vi "Slave - Latency Bmk - Queue.vi"() -> ()   [LabVIEW 2016]
uses:
  <vilib>/Utility/error.llb/DialogType.ctl
  <vilib>/Analysis/baseanly.llb/Mean (DBL).vi
  <vilib>/pximc/Initialize Writer Session (DBL).vi
  <vilib>/pximc/Initialize Reader Session (DBL).vi
  <vilib>/pximc/Connect (DBL).vi
  <vilib>/pximc/Write (DBL).vi
  <vilib>/pximc/Read (DBL).vi
  <vilib>/pximc/nipximc.lvlib
  <vilib>/Analysis/NI_AALBase.lvlib
panel:
  out "size(s) 2":i32
  out "size(s)":i32
  out "Avg Elapsed Time 2":dbl
  out "Value Change Timestamp 2":u32 caption="Tick Count(uSec)"
  out "Instant Elapsed Time 2":i32
  out "Avg Elapsed Time":dbl
  out "Instant Elapsed Time":i32
  out "Value Change Timestamp":u32 caption="Tick Count(uSec)"
  in  "Node 1 Reader Connection ID":u16=4
  in  "Reader Interface Node 2":tag="PXIMC2" caption="interface"
  in  "Node 2 Writer Connection ID":u16=3
  in  "Writer Interface Node 2":tag="PXIMC2" caption="interface"
  out "Stopped?":bool
  in  "Node 1 Writer Connection ID":u16=1
  in  "Node 1 Writer Interface":tag="PXIMC2" caption="interface"
  in  "Stop Button":bool
  in  "Node 1 Reader Interface":tag="PXIMC2" caption="interface"
  in  "Buffer Size":u64=250000 caption="buffer size"
  in  "Connection Timeout (s)":dbl=60.0 caption="timeout in seconds (-1)"
  in  "Node 1 Reader Connection ID":u16=2
  # "Node 1"
  # "Node 2"
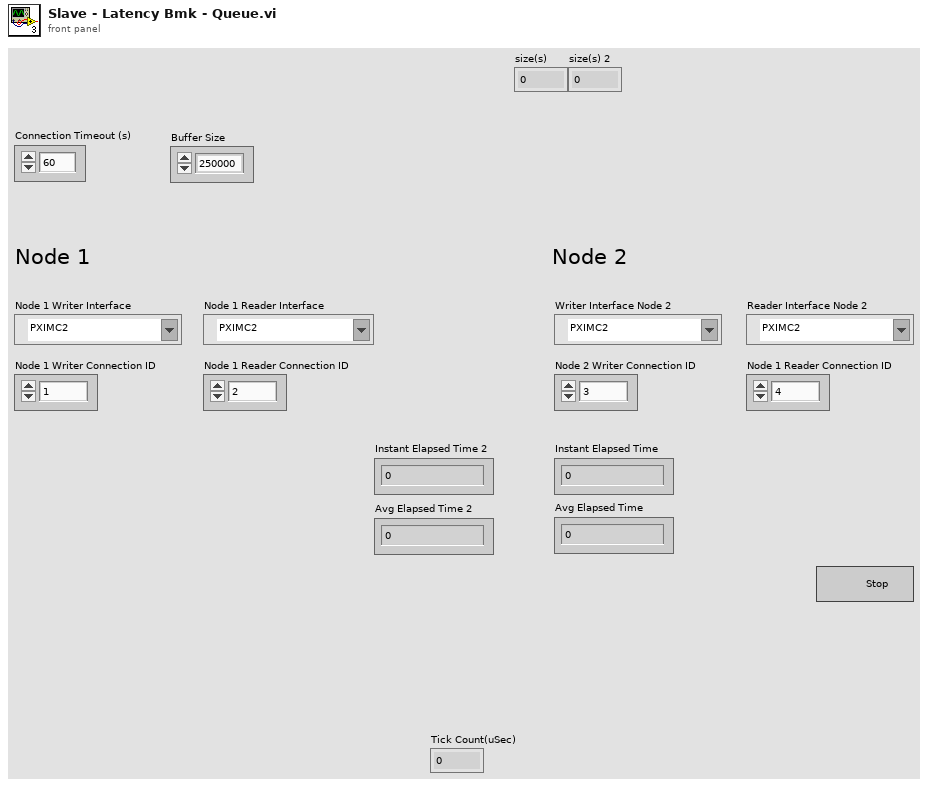
[diagram p1: front panel]
types:
  T1 = typedef "DialogType.ctl" = u16
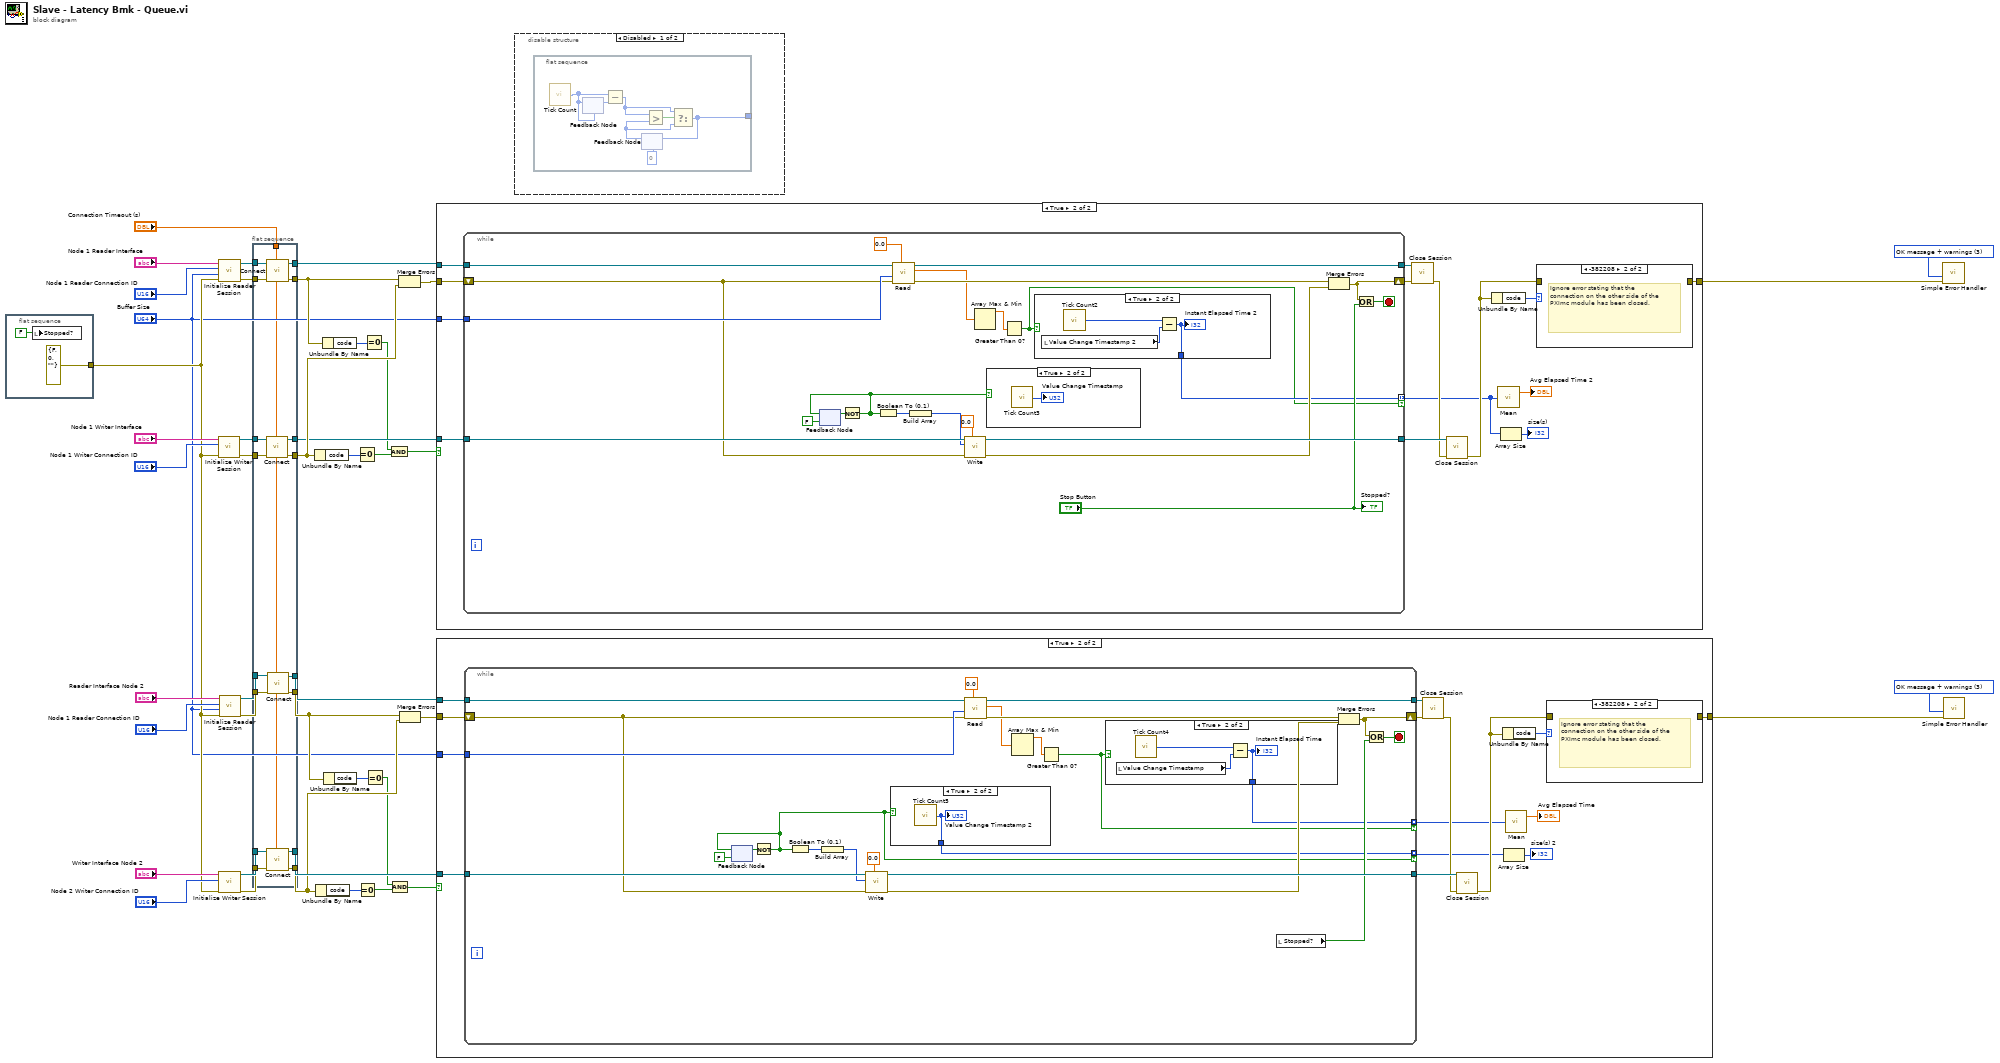
[diagram p0: block diagram]
diagram:
  w10 = T1 3 items=["no dialog", "OK message", "continue or stop message", "OK message + warnings", "continue/stop + warnings"] ("type of dialog (OK msg:1)")
  w37 = T1 3 items=["no dialog", "OK message", "continue or stop message", "OK message + warnings", "continue/stop + warnings"] ("type of dialog (OK msg:1)")
  n1 = flat-sequence {
    tunnel: [errorcluster {"status"=FALSE, "code"=0, "source"=""} ("error constant")] -> w3
    frame #0 {
      n2 = local write "Stopped?"(FALSE ("Stopped?")) -> ()
    }
  }
  n3 = call-poly <vilib>:"Initialize Writer Session.vi"("error in (no error)"=w3, "connection id (1)"="Node 1 Writer Connection ID", "interface"="Node 1 Writer Interface") -> ("error out"=w35:errorcluster, "session out"=w34:refnum<k21>)  [unwired: 7 in]
  n4 = call-poly <vilib>:"Initialize Reader Session.vi"("error in (no error)"=w3, "buffer size"="Buffer Size", "writer's connection id (1)"="Node 1 Reader Connection ID", "interface"="Node 1 Reader Interface") -> ("error out"=w41:errorcluster, "session out"=w42:refnum<k21>)  [unwired: 6 in]
  n5 = call-poly <vilib>:"Initialize Writer Session.vi"("error in (no error)"=w3, "connection id (1)"="Node 2 Writer Connection ID", "interface"="Writer Interface Node 2") -> ("error out"=w12:errorcluster, "session out"=w13:refnum<k21>)  [unwired: 7 in]
  n6 = call-poly <vilib>:"Initialize Reader Session.vi"("error in (no error)"=w3, "buffer size"="Buffer Size", "writer's connection id (1)"="Node 1 Reader Connection ID", "interface"="Reader Interface Node 2") -> ("error out"=w6:errorcluster, "session out"=w5:refnum<k21>)  [unwired: 6 in]
  n7 = flat-sequence {
    tunnel: w42 -> [w62]
    tunnel: w41 -> [w61]
    tunnel: [w60] -> w40
    tunnel: w35 -> [w59]
    tunnel: w34 -> [w58]
    tunnel: [w57] -> w28
    tunnel: [w56] -> w27
    tunnel: "Connection Timeout (s)" -> [w46]
    tunnel: [w55] -> w25
    tunnel: [w54] -> w22
    tunnel: [w53] -> w21
    tunnel: [w52] -> w20
    tunnel: w13 -> [w51]
    tunnel: w12 -> [w50]
    tunnel: [w49] -> w7
    tunnel: w6 -> [w48]
    tunnel: w5 -> [w47]
    frame #0 {
      n8 = call-poly <vilib>:"Connect.vi"("timeout in seconds (-1)"=w46, "error in (no error)"=w59, "session in"=w58) -> ("error out"=w56:errorcluster, "session out"=w55:refnum<k21>)  [unwired: 7 in]
      n9 = call-poly <vilib>:"Connect.vi"("timeout in seconds (-1)"=w46, "error in (no error)"=w61, "session in"=w62) -> ("error out"=w57:errorcluster, "session out"=w60:refnum<k21>)  [unwired: 7 in]
      n10 = call-poly <vilib>:"Connect.vi"("timeout in seconds (-1)"=w46, "error in (no error)"=w50, "session in"=w51) -> ("error out"=w53:errorcluster, "session out"=w54:refnum<k21>)  [unwired: 7 in]
      n11 = call-poly <vilib>:"Connect.vi"("timeout in seconds (-1)"=w46, "error in (no error)"=w48, "session in"=w47) -> ("error out"=w52:errorcluster, "session out"=w49:refnum<k21>)  [unwired: 7 in]
    }
  }
  n12 = Unbundle By Name(w27) -> ("code"=w32:i32)
  n13 = Unbundle By Name(w21) -> ("code"=w15:i32)
  n14 = Unbundle By Name(w28) -> ("code"=w38:i32)
  n15 = Unbundle By Name(w20) -> ("code"=w9:i32)
  n16 = Equal To 0?(x=w32) -> (x = 0?=w30:bool)
  n17 = Equal To 0?(x=w15) -> (x = 0?=w18:bool)
  n18 = Equal To 0?(x=w38) -> (x = 0?=w1:bool)
  n19 = Equal To 0?(x=w9) -> (x = 0?=w17:bool)
  n20 = And(x=w1, y=w30) -> (x .and. y?=w31:bool)
  n21 = And(x=w17, y=w18) -> (x .and. y?=w16:bool)
  n22 = Merge Errors(w28, w27) -> (w29:errorcluster)
  n23 = Merge Errors(w20, w21) -> (w19:errorcluster)
  n24 = case shown="True" w31 {
    tunnel: w29 -> [w63 w77]
    tunnel: w40 -> [_ w76]
    tunnel: [w63 w74] -> w24
    tunnel: "Buffer Size" -> [_ w71]
    tunnel: w25 -> [_ w70]
    frame False {
      # "The connection was not successful for some reason."
    }
    frame True {
      n25 = while {
        tunnel: w76 -> [w99]
        tunnel: [w98] -> w75
        shift-right: [w91] -> w72
        shift-left: w77 -> [w82]
        tunnel: w71 -> [w97]
        tunnel: w70 -> [w96]
        tunnel: [w95] -> w69
        tunnel: [w79] -> w65 mode=indexing if=w78
        stop <- w92 stop-if-true
        n26 = feedback #1(FALSE) -> (w84:bool)
        n27 = Not(x=w84) -> (.not. x?=w83:bool)
        n28 = feedback-in #1(w83) -> ()
        n29 = Boolean To (0,1)(Boolean=w83) -> (0, 1=w86:i16)
        n30 = call-poly <vilib>:"Read.vi"("timeout in seconds (5)"=0.0, "error in (no error)"=w82, "number of elements"=w97, "session in"=w99) -> ("error out"=w94:errorcluster, "data"=w80:dbl[], "session out"=w98:refnum<k21>)  [unwired: 5 in]
        n31 = Build Array(w86) -> (w87:i16[])
        n32 = call-poly <vilib>:"Write.vi"("timeout in seconds (5)"=0.0, "error in (no error)"=w82, "data"=w87, "session in"=w96) -> ("error out"=w93:errorcluster, "session out"=w95:refnum<k21>)  [unwired: 5 in, 1 out]
        n33 = Array Max & Min(array=w80) -> (max value=w81:dbl)  [unwired: 3 out]
        n34 = case shown="True" w83 {
          frame False {
          }
          frame True {
            n35 = call "Tick Count3"() -> ("Tick Count(uSec)"=→"Value Change Timestamp":u32)
          }
        }
        n36 = Greater Than 0?(x=w81) -> (x > 0?=w78:bool)
        n37 = case shown="True" w78 {
          tunnel: [_ w100] -> w79
          frame False {
          }
          frame True {
            n38 = local read "Value Change Timestamp 2"() -> (w102:u32)
            n39 = call "Tick Count2"() -> ("Tick Count(uSec)"=w101:u32)
            n40 = Subtract(x=w101, y=w102) -> (x-y=w100:u32)
            "Instant Elapsed Time 2" <- w100
          }
        }
        n41 = Merge Errors(w94, w93) -> (w91:errorcluster)
        n42 = Or(x=w91, y="Stop Button") -> (x .or. y?=w92:bool)
        "Stopped?" <- "Stop Button"
      }
      n43 = call <vilib>:"Close Session.vi"("error in (no error)"=w72, "session in"=w75) -> ("error out"=w68:errorcluster)  [unwired: 9 in]
      n44 = call <vilib>:"Close Session.vi"("error in (no error)"=w68, "session in"=w69) -> ("error out"=w67:errorcluster)  [unwired: 9 in]
      n45 = Unbundle By Name(w67) -> ("code"=w73:i32)
      n46 = call-poly <vilib>:"Mean.vi"("X"=w65) -> ("mean"=→"Avg Elapsed Time 2":dbl)  [unwired: 1 out]
      n47 = Array Size(array=w65) -> (size(s)=→"size(s)":i32)
      n48 = case shown="-382208" w73 {
        tunnel: w67 -> [w104 _]
        tunnel: [w104 _] -> w74
        frame 0, Default {
        }
        frame -382208 {
          # "Ignore error stating that the connection on the other side of the PXImc module has been closed."
        }
      }
    }
  }
  n49 = case shown="True" w16 {
    tunnel: w19 -> [w105 w120]
    tunnel: w7 -> [_ w119]
    tunnel: [w105 w117] -> w23
    tunnel: "Buffer Size" -> [_ w114]
    tunnel: w22 -> [_ w113]
    frame False {
      # "The connection was not successful for some reason."
    }
    frame True {
      n50 = while {
        tunnel: w119 -> [w143]
        tunnel: [w142] -> w118
        shift-right: [w135] -> w115
        shift-left: w120 -> [w124]
        tunnel: w114 -> [w141]
        tunnel: w113 -> [w140]
        tunnel: [w139] -> w112
        tunnel: [w131] -> w109 mode=indexing if=w130
        tunnel: [w122] -> w107 mode=indexing if=w121
        stop <- w136 stop-if-true
        n51 = feedback #2(FALSE) -> (w129:bool)
        n52 = Not(x=w129) -> (.not. x?=w121:bool)
        n53 = feedback-in #2(w121) -> ()
        n54 = Boolean To (0,1)(Boolean=w121) -> (0, 1=w127:i16)
        n55 = Build Array(w127) -> (w126:i16[])
        n56 = call-poly <vilib>:"Write.vi"("timeout in seconds (5)"=0.0, "error in (no error)"=w124, "data"=w126, "session in"=w140) -> ("error out"=w137:errorcluster, "session out"=w139:refnum<k21>)  [unwired: 5 in, 1 out]
        n57 = case shown="True" w121 {
          tunnel: [_ w144] -> w122
          frame False {
          }
          frame True {
            n58 = call "Tick Count5"() -> ("Tick Count(uSec)"=w144:u32)
            "Value Change Timestamp 2" <- w144
          }
        }
        n59 = call-poly <vilib>:"Read.vi"("timeout in seconds (5)"=0.0, "error in (no error)"=w124, "number of elements"=w141, "session in"=w143) -> ("error out"=w138:errorcluster, "data"=w125:dbl[], "session out"=w142:refnum<k21>)  [unwired: 5 in]
        n60 = Array Max & Min(array=w125) -> (max value=w123:dbl)  [unwired: 3 out]
        n61 = Greater Than 0?(x=w123) -> (x > 0?=w130:bool)
        n62 = case shown="True" w130 {
          tunnel: [_ w145] -> w131
          frame False {
          }
          frame True {
            n63 = local read "Value Change Timestamp"() -> (w147:u32)
            n64 = call "Tick Count4"() -> ("Tick Count(uSec)"=w146:u32)
            n65 = Subtract(x=w146, y=w147) -> (x-y=w145:u32)
            "Instant Elapsed Time" <- w145
          }
        }
        n66 = local read "Stopped?"() -> (w134:bool)
        n67 = Merge Errors(w138, w137) -> (w135:errorcluster)
        n68 = Or(x=w135, y=w134) -> (x .or. y?=w136:bool)
      }
      n69 = call <vilib>:"Close Session.vi"("error in (no error)"=w115, "session in"=w118) -> ("error out"=w111:errorcluster)  [unwired: 9 in]
      n70 = call <vilib>:"Close Session.vi"("error in (no error)"=w111, "session in"=w112) -> ("error out"=w110:errorcluster)  [unwired: 9 in]
      n71 = Unbundle By Name(w110) -> ("code"=w116:i32)
      n72 = Array Size(array=w107) -> (size(s)=→"size(s) 2":i32)
      n73 = call-poly <vilib>:"Mean.vi"("X"=w109) -> ("mean"=→"Avg Elapsed Time":dbl)  [unwired: 1 out]
      n74 = case shown="-382208" w116 {
        tunnel: w110 -> [w148 _]
        tunnel: [w148 _] -> w117
        frame 0, Default {
        }
        frame -382208 {
          # "Ignore error stating that the connection on the other side of the PXImc module has been closed."
        }
      }
    }
  }
  n75 = disable-structure shown="Disabled" {
    frame Disabled {
      n76 = flat-sequence {
        tunnel: [w149] -> _
        frame #0 {
          n77 = call "Tick Count"() -> ("Tick Count(uSec)"=w150:u32)
          n78 = feedback #3(w150) -> (w154:u32)
          n79 = feedback-in #3(w150) -> ()
          n80 = Subtract(x=w150, y=w154) -> (x-y=w155:u32)
          n81 = feedback #4(u32 0) -> (w151:u32)
          n82 = Greater?(x=w155, y=w151) -> (0:w152:bool)
          n83 = Select(t=w155, s=w152, f=w151) -> (s? t:f=w149:u32)
          n84 = feedback-in #4(w149) -> ()
        }
      }
    }
    frame Enabled {
    }
  }
  n85 = call <vilib>:"Simple Error Handler.vi"("type of dialog (OK msg:1)"=w37, "error in (no error)"=w24) -> ()  [unwired: 3 in, 5 out]
  n86 = call <vilib>:"Simple Error Handler.vi"("type of dialog (OK msg:1)"=w10, "error in (no error)"=w23) -> ()  [unwired: 3 in, 5 out]
